vi "UHR-Fleezers Control (fpga) - 9.2.vi"() -> ()   [LabVIEW 2009]
doc: "UHR-Fleezers Instrument Control Code (fpga)"
uses:
  <vilib>/Platform/TimedLoop/XDataNode/XDataNode.xnode
  <vilib>/Platform/TimedLoop/XDataNode/loadlvalarms.vi
  <vilib>/Platform/TimedLoop/XDataNode/timing_clust.ctl
  <vilib>/Platform/TimedLoop/XDataNode/nitl_modes.ctl
  <vilib>/Platform/TimedLoop/XDataNode/wakeup.ctl
  <vilib>/eio/EIONode/EIONode.xnode
  <vilib>/rvi/eio/nirviEIOImplementation/nirviEIOImplementation.xnode
  <vilib>/rvi/eio/common/nirviEmuTemplateMethod_noerrors.vi
  <vilib>/rvi/eio/common/nirviEmuClasses.ctl
  <vilib>/eio/EIOMethodNode/EIOMethodNode.xnode
  <vilib>/rvi/eio/nirviEIOMethodImplementation/nirviEIOMethodImplementation.xnode
  <vilib>/rvi/DataTransferAndStorage/Container/XNode/niFpgaContainer.xnode
  <vilib>/rvi/interface/RandomDataEmulation/niFpgaRandomDataHandleErrors.vi
  <vilib>/rvi/interface/RandomDataEmulation/nirviRandomDataFPGAFIFO.vi
  <vilib>/rvi/DataTransferAndStorage/Container/Common/niFpgaContainerMethod.ctl
  <vilib>/rvi/DataTransferAndStorage/Container/Common/niFpgaTransferTypeControl.ctl
  <vilib>/Platform/TimedLoop/XDataNode/XDNodeRunTimeDep.lvlib
panel:
  in  "Tab Control":T1(tab)=enum."APD Counting"
  in  "AI Averages":u16=1 min=1 step=1
  in  "AI1 Sets to FIFO":T2={"Set 1"=TRUE, "Set 2"=TRUE, "Set 3"=FALSE}
  in  "N of AI1 Int Acq Sets":i16=2 min=1 max=3 step=1
  out "Number of AI channels":i16
  out "AI Late Counter":u32
  in  "ai count":u32=400
  out "AI late?":bool
  in  "+ phase":bool
  in  "Phase count adjustment":i16
  out "Relative phase":i16
  in  "DMA buffer timeout":i32
  in  "AI to FIFO":bool
  in  "Tab Control 2":T3(tab)
  in  "Swap F1 and F2":bool
  in  "Freq or Amp switch first":bool=TRUE
  in  "Cont. Scan":bool
  in  "Abort scan":bool
  in  "Cycles per step":u64
  in  "Scan BD":bool
  in  "Number of scans":u16
  in  "Scan steps":u64
  in  "Scan freq.  increment":i64
  out "Scanning":bool
  in  "Start scan":bool
  in  "OSK Bd 1":bool
  in  "Reset Bd 1":bool
  in  "RD":bool
  in  "PMODE":bool
  in  "OSK Bd 2":bool
  in  "Reset Bd 2":bool
  in  "Direct RF Box \nCommunication":bool
  in  "Data BD 2":u8 format="%08b"
  in  "Data BD 1":u8 format="%08b"
  in  "Address":u8 format="%02x"
  in  "Update Data":bool
  in  "FPGA Controls\n RF Box":bool
  in  "Number Interlace Cycles":u8=2 min=1 max=3
  in  "Interlace Off Parameters":u8=1 min=1 max=3
  in  "Interlace ON/OFF":bool
  out "DIO Relative phase":i16
  in  "Phase count adjustment (DIO)":i16
  in  "+ phase (DIO)":bool
  out "DIO Late Counter":u32
  out "DIO Late?":bool
  in  "DIO count 1 (ticks)":u32=400
  in  "DIO count 2 (ticks)":u32=400
  in  "DIO count 3 (ticks)":u32=400
  out "AI2 Y Sum Set 2":i16
  out "AI2 Y Sum Set 1":i16
  in  "FB Gains Set 1":T4={"proportional gain (Kc)"=10, "integral gain (Kc*Ts/Ti)"=5, "derivative gain (Kc*Td/Ts)"=0}
  in  "FB Setpoint Set 1":i16 min=0 step=1
  in  "FB Reset Set 1":bool
  in  "FB On/Off Set 1":bool
  in  "FB Reset Set 2":bool
  in  "FB On/Off Set 2":bool
  in  "FB Setpoint Set 2":i16 min=0 step=1
  in  "FB Gains Set 2":T4={"proportional gain (Kc)"=10, "integral gain (Kc*Ts/Ti)"=5, "derivative gain (Kc*Td/Ts)"=0}
  in  "FB output range 2":cluster{"output high":i16, "output low":i16}={"output high"=3000, "output low"=0}
  in  "FB output range 1":cluster{"output high":i16, "output low":i16}={"output high"=3000, "output low"=0}
  out "Scan I":u64
  in  "Amp switch delay":u16=5
  in  "Freq switch delay":u16
  in  "BD 2 Amplitude 1":u16
  in  "BD 1 Amplitude 1":u16
  in  "BD 2 Frequency 1":u64
  in  "BD 1 Frequency 1":u64
  in  "BD 2 Amplitude 2":u16
  in  "BD 1 Amplitude 2":u16
  in  "BD 2 Frequency 2":u64
  in  "BD 1 Frequency 2":u64
  in  "BD 2 Amplitude 3":u16
  in  "BD 1 Amplitude 3":u16
  in  "BD 2 Frequency 3":u64
  in  "BD 1 Frequency 3":u64
  out "Numeric":i32
  out "AO2 2":i16
  out "AO1 2":i16
  in  "1D or 2D Scan?":bool
  in  "Abort scan (MCL)":bool
  in  "MCL Scan Axis":bool
  in  "Cont. Scan (MCL)":bool
  out "Scan I (MCL)":u64
  in  "Number of scans (MCL)":u16
  out "Scanning MCL":bool
  in  "Scan steps (MCL)":u64
  in  "Cycles per step (MCL)":u64
  in  "Scan freq.  increment (MCL)":i16
  in  "Start scan (MCL)":bool
  in  "AO2":i16
  in  "AO1":i16
  out "MCL Late Counter":u32
  out "MCL Late?":bool
  in  "MCL count":u32=800
  out "MCL Relative Phase":i16
  in  "Phase count adjustment (MCL)":i16
  in  "+ phase (MCL)":bool
  in  "APD2 Trigger on Edge?":bool=TRUE
  in  "APD1 Trigger on Edge?":bool=TRUE
  in  "APD Gate Operating Mode":u8 max=2 step=1
  in  "Invert APD Gate":bool
  in  "APD Gate OFF Count":u32=100
  in  "APD Gate ON Count":u32=300
  out "APD Gate Late Counter":u32
  out "APD Gate Late?":bool
  out "APD Gate Relative Phase":i16
  in  "Phase count adjustment (APD Gate)":i16
  in  "+ phase (APD Gate)":bool
  out "APD 2 Counts 0":u32
  out "APD 2 Counts 1":u32
  out "APD 1 Counts 0":u32
  out "APD 1 Counts 1":u32
  out "APD out state":bool
  in  "APD 2 AO offset":i16
  in  "APD 1 AO offset":i16
  in  "APD 2 AO scale factor":i16=1
  in  "APD 1 AO scale factor":i16=1
  in  "APD to FIFO":bool
  in  "APD Acq Rate Count":u32=20000000
  out "APD Acq Late Counter":u32
  out "APD Acq Late?":bool
  out "APD Acq Relative Phase":i16
  in  "Phase Count Adjustment (APD Acq)":i16
  in  "+ phase (APD Acq)":bool
  in  "Green Filter Flipper":bool
  out "Green FB Signals":T5
  in  "Green FB Count":u32=1200
  out "Green Late Counter":u32
  out "Green FB Late?":bool
  out "Green FB Relative Phase":i16
  in  "Phase count adjustment (Green FB)":i16=10
  in  "+ phase (Green FB)":bool
  out "Green FB Sum":i16
  in  "Green int current ON count adj":u32=150
  in  "Current Out":u16=30000
  in  "Green FB On/Off":bool
  in  "Green FB Setpoint":i16=250 min=0 step=1
  in  "Green FB Gains":T4={"proportional gain (Kc)"=10, "integral gain (Kc*Ts/Ti)"=5, "derivative gain (Kc*Td/Ts)"=0}
  in  "Green FB Reset":bool
  in  "Operating Mode 2":u8=2 max=2 step=1
  in  "Invert GI 2":bool
  in  "Green interlace OFF count 2":u32=900
  in  "Green interlace ON count 2":u32=300
  out "GI Late Counter 2":u32
  out "GI Late? 2":bool
  out "GI Relative phase 2":i16
  in  "Phase count adjustment (GI) 2":i16=20
  in  "+ phase (GI) 2":bool
  in  "Green interlace OFF count":u32=100
  out "GI Relative phase":i16
  in  "Phase count adjustment (GI)":i16
  in  "+ phase (GI)":bool
  out "GI Late?":bool
  in  "Green interlace ON count":u32=300
  out "GI Late Counter":u32
  in  "Invert GI":bool
  in  "Operating Mode":u8 max=2 step=1
  in  "Connector0/DIO9":bool
  in  "Connector1/DIO32":bool
  in  "Connector1/DIO33":bool
  in  "Connector1/DIO34":bool
  in  "Chassis2/Mod4/AO1":u16
  in  "Extra DO Counts":u32=40000
  # "Only one of these can be on\nat a time:"
  # "Raster Scan AOD"
  # "1 (X)"
  # "2 (Y)"
  # "IR Intensity Feedback (RF BD 1)"
  # "AO1 (Y)"
  # "2D"
  # "1D"
  # "AO2 (X)"
  # "APD AO for aligning"
  # "Detection Loop"
  # "Green fluorescent laser digital gate interlacing loop"
  # "0 Forced ON\n1 Forced OFF\n2 Interlacing"
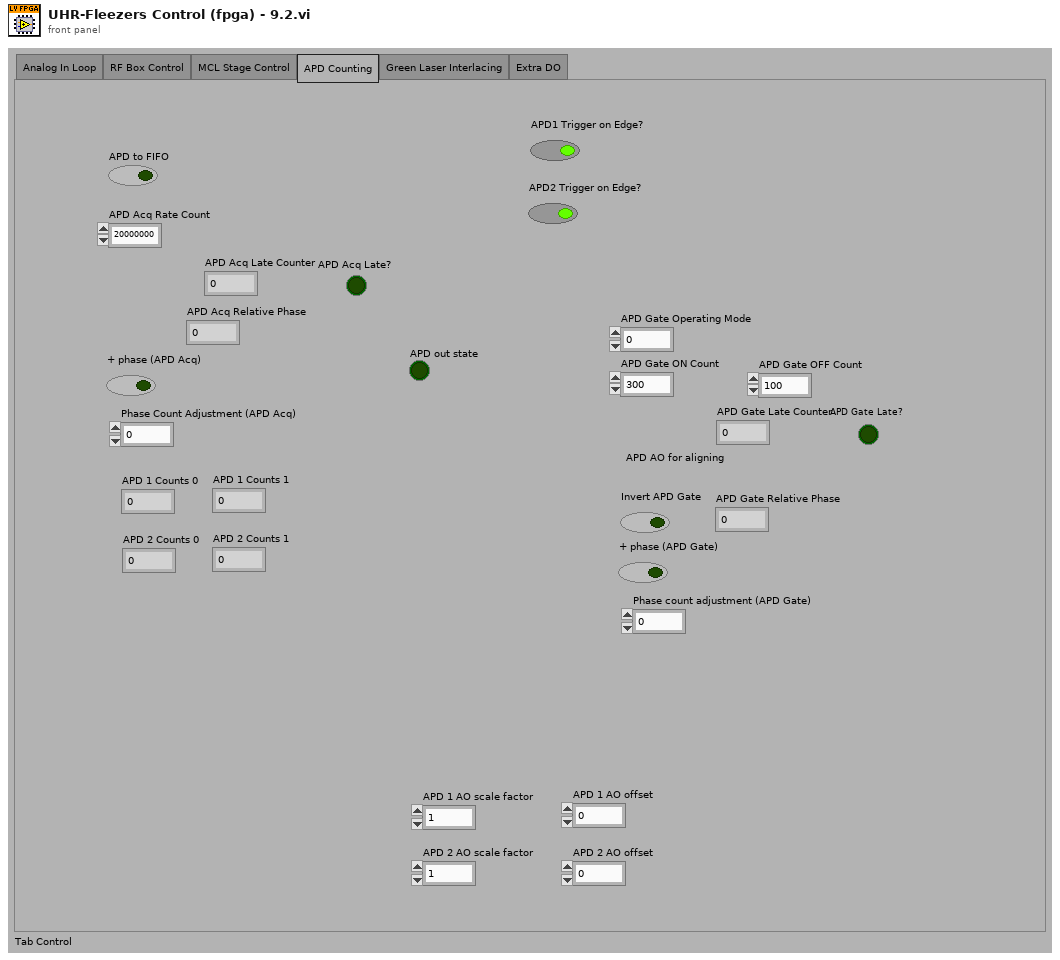
[diagram p1: front panel]
types:
  T1 = enum32{"Analog In Loop", "RF Box Control", "MCL Stage Control", "APD Counting", "Green Laser Interlacing", "Extra DO"}
  T2 = cluster{"Set 1":bool, "Set 2":bool, "Set 3":bool}
  T3 = enum32{"Controls", "Interlacing Frequency and Amplitude Values"}
  T4 = cluster{"proportional gain (Kc)":i16, "integral gain (Kc*Ts/Ti)":i16, "derivative gain (Kc*Td/Ts)":i16}
  T5 = cluster{"Green FB Ch 0":i16, "Green FB Ch 1":i16, "Green FB Ch 2":i16}
  T6 = typedef "nirviEmuClasses.ctl" = enum16{"IO Read", "IO Write", "Method", "Property Read", "Property Write"}
  T7 = typedef "XDNodeRunTimeDep.lvlib/timing_clust.ctl" = cluster{"Expected End [f-1]":u64, "Actual End [f-1]":u64, "Finished Late? [f-1]":bool, "Expected End [i-1]":u64, "Actual End [i-1]":u64, "Finished Late? [i-1]":bool, "Expected Start [i]":u64, "Actual Start [i]":u64, "Expected Start [f]":u64, "Actual Start [f]":u64, "Source Name":string, "Structure Name":string, "Period":i64, "Deadline":i64, "Offset":i64, "Start":i64, "Priority":i32, "Timeout":i32, "Mode":T8, "Wakeup Reason":T9, "Error":errorcluster, "Source Type":string, "Secondary Source Type":string, "Global End Time":u64, "Global Start Time":u64, "Frame Duration":u64, "Iteration Duration":u64, "Assigned CPU":i32, "I/O Scan Engine Mode":u32}
  T8 = typedef "XDNodeRunTimeDep.lvlib/nitl_modes.ctl" = enum32{"No Change", "Process missed periods, maintain original phase", "Discard missed periods, maintain original phase", "Process missed periods, ignore original phase", "Discard missed periods, ignore original phase"}
  T9 = typedef "XDNodeRunTimeDep.lvlib/wakeup.ctl" = enum32{"Normal", "Aborted", "Asynchronous wakeup", "Timing source error", "Timed loop error", "Timeout"}
  T10 = cluster{"Chassis2/Mod1/AI0":i16, "Chassis2/Mod1/AI1":i16, "Chassis2/Mod1/AI2":i16}
  T11 = typedef "niFpgaContainerMethod.ctl" = enum16{"Write", "Read", "Clear", "Get Number of Elements to Write", "Get Number of Elements to Read", "Enable", "Disable", "Flush and Disable", "Get Stream State"}
  T12 = typedef "niFpgaTransferTypeControl.ctl" = enum16{"Target-Scoped", "Host to Target - DMA", "Target to Host - DMA", "Peer to Peer Reader", "Peer to Peer Writer", "Bidirectional"}
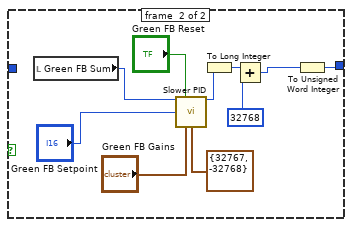
[diagram p2: hidden frame]
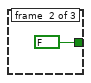
[diagram p3: hidden frame]
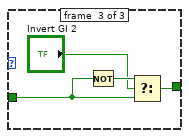
[diagram p4: hidden frame]
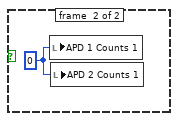
[diagram p5: hidden frame]
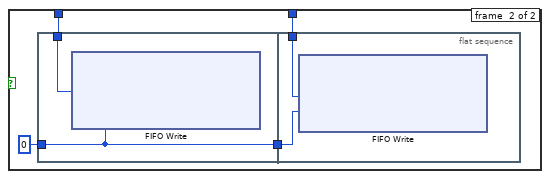
[diagram p6: hidden frame]
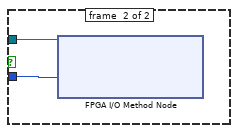
[diagram p7: hidden frame]
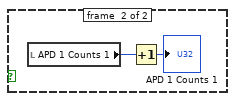
[diagram p8: hidden frame]
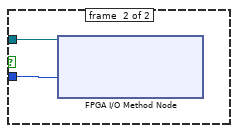
[diagram p9: hidden frame]
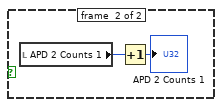
[diagram p10: hidden frame]
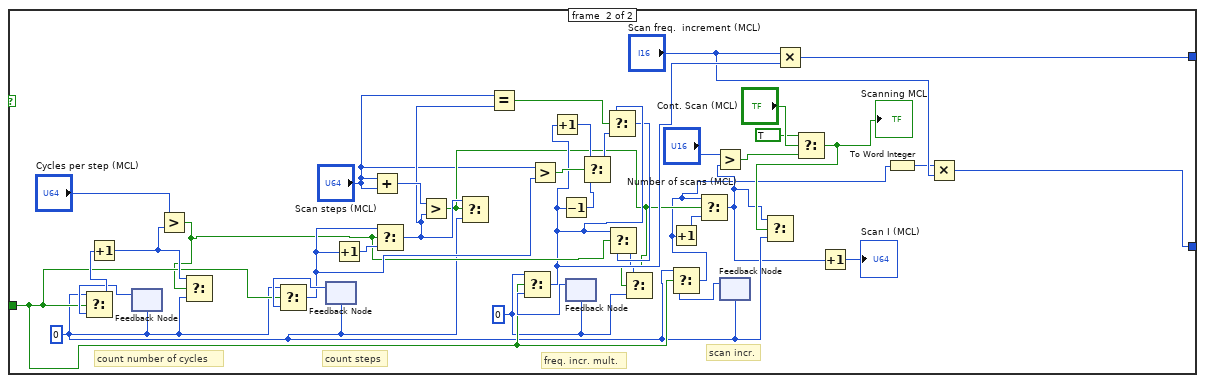
[diagram p11: hidden frame]
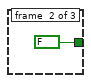
[diagram p12: hidden frame]
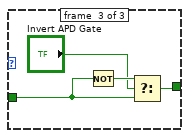
[diagram p13: hidden frame]
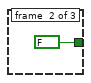
[diagram p14: hidden frame]
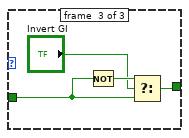
[diagram p15: hidden frame]
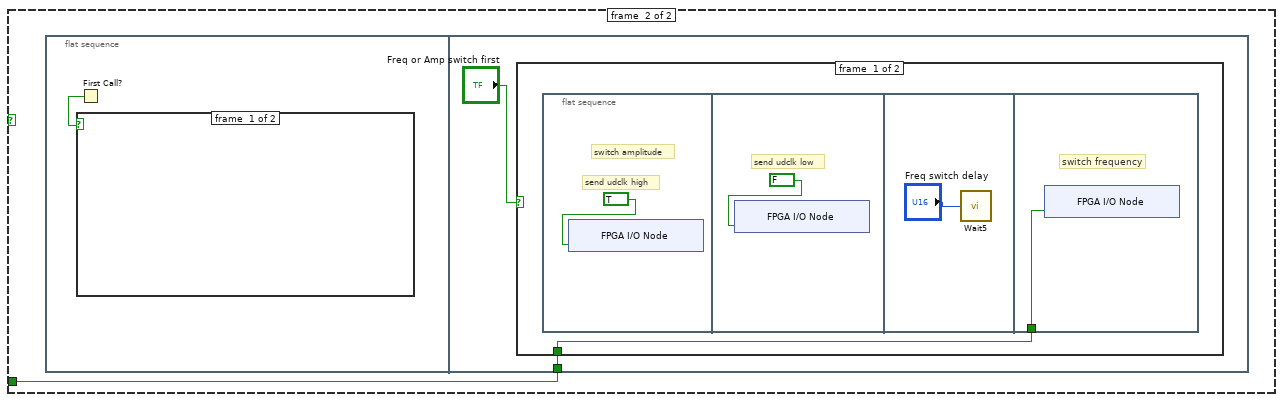
[diagram p16: hidden frame]
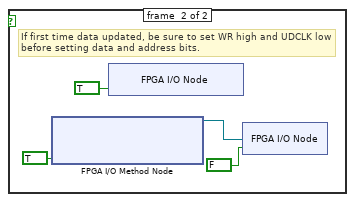
[diagram p17: hidden frame]
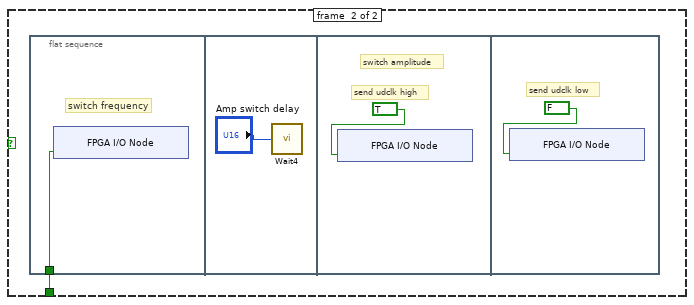
[diagram p18: hidden frame]
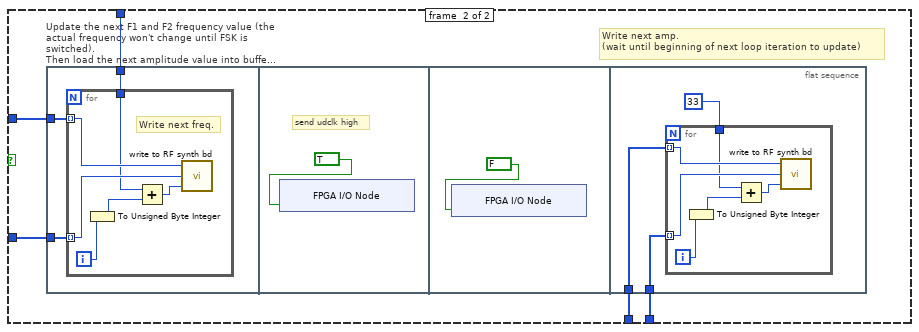
[diagram p19: hidden frame]
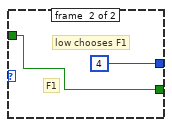
[diagram p20: hidden frame]
diagram:
  # "timing array current index"
  # "timing array"
  # "timing counter (phase adjusted here)"
  # "late counter"
  n1 = flat-sequence "FPGA initialization to do before running any of the loops" {
    tunnel: [u32 0 ("DIO count 3 (ticks)")] -> w1
    tunnel: [w10] -> _
    frame #0 {
      # "This is a kludge to let host programs know how many channels of data are in the DMA stream.  Set by hand."
      # "Start up expansion chassis early\nto avoid delays later"
      # "This pin controls udclk on the RF boards.\nWhen initially configuring the boards, this pin needs to be\nconfigured as a high impedance input.  Later it will be switched\nto an output."
      # "Initial setting of DIO data and \naddress to low (before reset).  \nThis needs to happen before the other\ncontrol method loops execute."
      n2 = xnode "FPGA I/O Node"("Chassis2/Mod4/AO0"=u16 0) -> ("Chassis2/Mod1/AI0"=w10:i16)  [unwired: 2 in, 2 out]
      n3 = xnode "FPGA I/O Method Node"("Enable"=FALSE) -> ()  [unwired: 1 in, 1 out]
      n4 = xnode "FPGA I/O Node"("Connector1/DIO0"=FALSE, "Connector1/DIO1"=FALSE, "Connector1/DIO2"=FALSE, "Connector1/DIO3"=FALSE, "Connector1/DIO4"=FALSE, "Connector1/DIO5"=FALSE, "Connector1/DIO6"=FALSE, "Connector1/DIO7"=FALSE, "Connector1/DIO8"=FALSE, "Connector1/DIO9"=FALSE, "Connector1/DIO10"=FALSE, "Connector1/DIO11"=FALSE, "Connector1/DIO12"=FALSE, "Connector1/DIO13"=FALSE, "Connector1/DIO15"=FALSE, "Connector1/DIO20"=FALSE, "Connector1/DIO21"=FALSE, "Connector1/DIO22"=FALSE, "Connector1/DIO23"=FALSE, "Connector1/DIO24"=FALSE, "Connector1/DIO25"=FALSE, "Connector1/DIO26"=FALSE, "Connector1/DIO27"=FALSE, "Connector1/DIO14"=FALSE) -> ()  [unwired: 24 in, 24 out]
      "Number of AI channels" <- i16 12 ("Number of AI channels")
    }
  }
  n5 = node-c288() -> (w3:T7)  [unwired: 1 in]
  n6 = local read "AO1"() -> (w5:i16)
  n7 = local read "AO2"() -> (w4:i16)
  n8 = timed-loop "RF box board DIO control: control bits" {
    timing: w3 -> [_]
    timing-out: [_] -> w2
    tunnel: [w393] -> _
    tunnel: w1 -> [w393]
    stop <- FALSE stop-if-true
    n9 = xnode "FPGA I/O Node"("Connector1/DIO16"="RD", "Connector1/DIO17"="PMODE", "Connector1/DIO18"="OSK Bd 1", "Connector1/DIO19"="Reset Bd 1", "Connector1/DIO28"="OSK Bd 2", "Connector1/DIO29"="Reset Bd 2") -> ()  [unwired: 6 in, 6 out]
  }
  n10 = while "APD 1 Counter" {
    tunnel: w1 -> [_]
    stop <- FALSE stop-if-true
    n11 = flat-sequence {
      frame #0 {
        n12 = case shown="False" "APD1 Trigger on Edge?" {
          tunnel: refnum<k21> "Connector0/DIO10" ("APD 1 DO") -> [w486 w511]
          tunnel: -1 ("Timeout") -> [w485 w510]
          frame #0 {
            n13 = xnode "FPGA I/O Method Node"("FPGA I/O In"=w486, "Timeout"=w485) -> ()  [unwired: 2 out]
          }
          frame #1 {
            n14 = xnode "FPGA I/O Method Node"("FPGA I/O In"=w511, "Timeout"=w510) -> ()  [unwired: 2 out]
          }
        }
      }
      frame #1 {
        n15 = local read "APD out state"() -> (w535:bool)
        n16 = case shown="False" w535 {
          frame #0 {
            n17 = local read "APD 1 Counts 0"() -> (w537:u32)
            n18 = Increment(x=w537) -> (x+1=→"APD 1 Counts 0":u32)
          }
          frame #1 {
            n19 = local read "APD 1 Counts 1"() -> (w539:u32)
            n20 = Increment(x=w539) -> (x+1=→"APD 1 Counts 1":u32)
          }
        }
      }
    }
  }
  n21 = while "APD 2 Counter" {
    tunnel: w1 -> [_]
    stop <- FALSE stop-if-true
    n22 = flat-sequence {
      frame #0 {
        n23 = case shown="False" "APD2 Trigger on Edge?" {
          tunnel: refnum<k21> "Connector0/DIO11" ("APD 2 DO") -> [w545 w570]
          tunnel: -1 ("Timeout") -> [w544 w569]
          frame #0 {
            n24 = xnode "FPGA I/O Method Node"("FPGA I/O In"=w545, "Timeout"=w544) -> ()  [unwired: 2 out]
          }
          frame #1 {
            n25 = xnode "FPGA I/O Method Node"("FPGA I/O In"=w570, "Timeout"=w569) -> ()  [unwired: 2 out]
          }
        }
      }
      frame #1 {
        n26 = local read "APD out state"() -> (w594:bool)
        n27 = case shown="False" w594 {
          frame #0 {
            n28 = local read "APD 2 Counts 0"() -> (w596:u32)
            n29 = Increment(x=w596) -> (x+1=→"APD 2 Counts 0":u32)
          }
          frame #1 {
            n30 = local read "APD 2 Counts 1"() -> (w598:u32)
            n31 = Increment(x=w598) -> (x+1=→"APD 2 Counts 1":u32)
          }
        }
      }
    }
  }
  n32 = while "APD Gating" {
    shift-right: [w602] -> _
    shift-left: w1 -> [w607]
    shift-right: [w601] -> _
    shift-left: FALSE -> [w599]
    stop <- FALSE stop-if-true
    n33 = flat-sequence {
      tunnel: w607 -> [w610]
      tunnel: [w611] -> w605
      tunnel: [w610] -> w603
      tunnel: [w609] -> w600
      tunnel: w599 -> [w609]
      tunnel: [w614] -> w606
      tunnel: w605 -> [w614]
      tunnel: [w613] -> w604
      tunnel: w603 -> [w613]
      tunnel: w600 -> [w612]
      tunnel: [w724] -> w602
      tunnel: w606 -> [w746]
      tunnel: w604 -> [w743]
      tunnel: [w729] -> w601
      frame #0 {
        n34 = call "Loop Timer7"("Count(Ticks)"=w610) -> ("Tick Count(Ticks)"=w611:u32)
      }
      frame #1 {
        # "Can switch 2 APDs\n(need 4 channels/APD)"
        n35 = xnode "FPGA I/O Node"("Connector0/DIO0"=w612, "Connector0/DIO1"=w612, "Connector0/DIO2"=w612, "Connector0/DIO3"=w612, "Connector0/DIO4"=w612, "Connector0/DIO5"=w612, "Connector0/DIO6"=w612, "Connector0/DIO7"=w612) -> ()  [unwired: 8 in, 8 out]
      }
      frame #2 {
        n36 = feedback #1(TRUE) -> (w732:bool)
        n37 = feedback #2(w746) -> (w745:u32)
        n38 = Not(x=w732) -> (.not. x?=w728:bool)
        n39 = Subtract(x=w746, y=w745) -> (x-y=w744:u32)
        n40 = Select(t="APD Gate ON Count", s=w728, f="APD Gate OFF Count") -> (s? t:f=w734:u32)
        n41 = Subtract(x=w744, y=w743) -> (x-y=w735:u32)
        n42 = Subtract(x=w734, y=w735) -> (x-y=w723:u32)
        n43 = Greater?(x=w735, y=u32 0) -> (0:w739:bool)
        "APD Gate Late?" <- w739
        n44 = Boolean To (0,1)(Boolean="+ phase (APD Gate)") -> (0, 1=w721:i16)
        n45 = Multiply(x=w721, y="Phase count adjustment (APD Gate)") -> (x*y=w719:i16)
        n46 = feedback #3(u32 0) -> (w741:u32)
        n47 = Increment(x=w741) -> (x+1=w740:u32)
        n48 = Select(t=w740, s=w739, f=w741) -> (s? t:f=w738:u32)
        "APD Gate Late Counter" <- w738
        n49 = Add(x=w723, y=w719) -> (x+y=w724:u32)
        n50 = feedback #4(i16 0) -> (w726:i16)
        n51 = Subtract(x=w726, y=w719) -> (x-y=w725:i16)
        "APD Gate Relative Phase" <- w725
        n52 = case shown="2" "APD Gate Operating Mode" {
          tunnel: [TRUE FALSE w752] -> w729
          tunnel: w732 -> [_ _ w749]
          frame #0 {
          }
          frame #1 {
          }
          frame #2 {
            n53 = Not(x=w749) -> (.not. x?=w751:bool)
            n54 = Select(t=w751, s="Invert APD Gate", f=w749) -> (s? t:f=w752:bool)
          }
        }
      }
    }
  }
  n55 = while "Control Additional IO (Green laser flip mount)" {
    stop <- FALSE stop-if-true
    n56 = xnode "FPGA I/O Node"("Connector0/DIO8"="Green Filter Flipper", "Connector0/DIO9"="Connector0/DIO9", "Connector1/DIO32"="Connector1/DIO32", "Connector1/DIO33"="Connector1/DIO33", "Connector1/DIO34"="Connector1/DIO34", "Chassis2/Mod4/AO1"="Chassis2/Mod4/AO1") -> ()  [unwired: 6 in, 6 out]
    n57 = call "Loop Timer2"("Count(Ticks)"="Extra DO Counts") -> ()  [unwired: 1 out]
  }
  n58 = while "Green excitation laser feedback measurement" {
    shift-right: [w827] -> _
    shift-left: w1 -> [w832]
    stop <- FALSE stop-if-true
    n59 = flat-sequence {
      tunnel: w832 -> [w834]
      tunnel: [w835] -> w830
      tunnel: [w834] -> w828
      tunnel: [w842] -> w831
      tunnel: w830 -> [w842]
      tunnel: [w841] -> w829
      tunnel: w828 -> [w841]
      tunnel: [w918] -> w827
      tunnel: w831 -> [w936]
      tunnel: w829 -> [w933]
      frame #0 {
        n60 = call "Loop Timer9"("Count(Ticks)"=w834) -> ("Tick Count(Ticks)"=w835:u32)
      }
      frame #1 {
        n61 = xnode "FPGA I/O Node"("Connector1/DIO35"=TRUE) -> ("Chassis2/Mod1/AI0"=w840:i16, "Chassis2/Mod1/AI1"=w839:i16, "Chassis2/Mod1/AI2"=w836:i16)  [unwired: 4 in, 4 out]
        "Green FB Sum" <- w836
        n62 = Bundle("Chassis2/Mod1/AI0"=w840, "Chassis2/Mod1/AI1"=w839, "Chassis2/Mod1/AI2"=w836) -> (→"Green FB Signals":T10)  [unwired: 1 out]
      }
      frame #2 {
        n63 = feedback #5(w936) -> (w935:u32)
        n64 = Subtract(x=w936, y=w935) -> (x-y=w934:u32)
        n65 = xnode "FPGA I/O Node"("Connector1/DIO35"=FALSE) -> ()  [unwired: 1 in, 1 out]
        n66 = Subtract(x=w934, y=w933) -> (x-y=w927:u32)
        n67 = Subtract(x="Green FB Count", y=w927) -> (x-y=w922:u32)
        n68 = Greater?(x=w927, y=u32 0) -> (0:w929:bool)
        "Green FB Late?" <- w929
        n69 = Boolean To (0,1)(Boolean="+ phase (Green FB)") -> (0, 1=w920:i16)
        n70 = Multiply(x=w920, y="Phase count adjustment (Green FB)") -> (x*y=w915:i16)
        n71 = feedback #6(u32 0) -> (w931:u32)
        n72 = Increment(x=w931) -> (x+1=w930:u32)
        n73 = Select(t=w930, s=w929, f=w931) -> (s? t:f=w928:u32)
        "Green Late Counter" <- w928
        n74 = Add(x=w922, y=w915) -> (x+y=w918:u32)
        n75 = feedback #7(i16 0) -> (w917:i16)
        n76 = Subtract(x=w917, y=w915) -> (x-y=w916:i16)
        "Green FB Relative Phase" <- w916
      }
    }
  }
  n77 = while "Green fluorescent laser interlacing (DO to IA 532 nm AOM ME amp)." {
    shift-right: [w952] -> _
    shift-left: w1 -> [w957]
    shift-right: [w951] -> _
    shift-left: FALSE -> [w949]
    stop <- FALSE stop-if-true
    n78 = flat-sequence {
      tunnel: w957 -> [w960]
      tunnel: [w961] -> w955
      tunnel: [w960] -> w953
      tunnel: [w959] -> w950
      tunnel: w949 -> [w959]
      tunnel: [w964] -> w956
      tunnel: w955 -> [w964]
      tunnel: [w963] -> w954
      tunnel: w953 -> [w963]
      tunnel: w950 -> [w962]
      tunnel: [w1004] -> w952
      tunnel: w956 -> [w1031]
      tunnel: w954 -> [w1028]
      tunnel: [w1014] -> w951
      frame #0 {
        n79 = call "Loop Timer4"("Count(Ticks)"=w960) -> ("Tick Count(Ticks)"=w961:u32)
      }
      frame #1 {
        n80 = xnode "FPGA I/O Node"("Connector1/DIO37"=w962, "Connector1/DIO38"=w962, "Connector1/DIO39"=w962) -> ()  [unwired: 3 in, 3 out]
      }
      frame #2 {
        n81 = feedback #8(w1031) -> (w1030:u32)
        n82 = Subtract(x=w1031, y=w1030) -> (x-y=w1029:u32)
        n83 = Subtract(x=w1029, y=w1028) -> (x-y=w1020:u32)
        n84 = Greater?(x=w1020, y=u32 0) -> (0:w1024:bool)
        "GI Late?" <- w1024
        n85 = Boolean To (0,1)(Boolean="+ phase (GI)") -> (0, 1=w1009:i16)
        n86 = Multiply(x=w1009, y="Phase count adjustment (GI)") -> (x*y=w1006:i16)
        n87 = feedback #9(u32 0) -> (w1026:u32)
        n88 = Increment(x=w1026) -> (x+1=w1025:u32)
        n89 = Select(t=w1025, s=w1024, f=w1026) -> (s? t:f=w1023:u32)
        "GI Late Counter" <- w1023
        n90 = feedback #10(i16 0) -> (w1007:i16)
        n91 = Subtract(x=w1007, y=w1006) -> (x-y=w1005:i16)
        "GI Relative phase" <- w1005
        n92 = feedback #11(TRUE) -> (w1017:bool)
        n93 = case shown="2" "Operating Mode" {
          tunnel: [TRUE FALSE w1037] -> w1014
          tunnel: w1017 -> [_ _ w1034]
          frame #0 {
          }
          frame #1 {
          }
          frame #2 {
            n94 = Not(x=w1034) -> (.not. x?=w1036:bool)
            n95 = Select(t=w1036, s="Invert GI", f=w1034) -> (s? t:f=w1037:bool)
          }
        }
        n96 = Not(x=w1017) -> (.not. x?=w1013:bool)
        n97 = Select(t="Green interlace ON count", s=w1013, f="Green interlace OFF count") -> (s? t:f=w1019:u32)
        n98 = Subtract(x=w1019, y=w1020) -> (x-y=w1010:u32)
        n99 = Add(x=w1010, y=w1006) -> (x+y=w1004:u32)
      }
    }
  }
  n100 = while "Green fluorescent laser interlacing (Current to IA 532 nm AOM ME amp)." {
    shift-right: [w1043] -> _
    shift-left: w1 -> [w1046]
    shift-right: [w1040] -> _
    shift-left: w1 -> [w1038]
    stop <- FALSE stop-if-true
    n101 = flat-sequence {
      tunnel: w1046 -> [w1049]
      tunnel: [w1050] -> w1045
      tunnel: [w1049] -> w1044
      tunnel: [w1048] -> w1039
      tunnel: w1038 -> [w1048]
      tunnel: [w1053] -> w1042
      tunnel: w1045 -> [w1053]
      tunnel: [w1052] -> w1041
      tunnel: w1044 -> [w1052]
      tunnel: w1039 -> [w1051]
      tunnel: [w1066] -> w1043
      tunnel: [w1084] -> w1040
      tunnel: w1042 -> [w1103]
      tunnel: w1041 -> [w1100]
      frame #0 {
        n102 = call "Loop Timer10"("Count(Ticks)"=w1049) -> ("Tick Count(Ticks)"=w1050:u32)
      }
      frame #1 {
        n103 = xnode "FPGA I/O Node"("Chassis2/Mod4/AO0"=w1051) -> ()  [unwired: 1 in, 1 out]
      }
      frame #2 {
        n104 = Subtract(x="Green interlace OFF count 2", y="Green int current ON count adj") -> (x-y=w1076:u32)
        n105 = feedback #12(w1103) -> (w1102:u32)
        n106 = Add(x="Green int current ON count adj", y="Green interlace ON count 2") -> (x+y=w1077:u32)
        n107 = Subtract(x=w1103, y=w1102) -> (x-y=w1101:u32)
        n108 = Subtract(x=w1101, y=w1100) -> (x-y=w1092:u32)
        n109 = Greater?(x=w1092, y=u32 0) -> (0:w1096:bool)
        "GI Late? 2" <- w1096
        n110 = Boolean To (0,1)(Boolean="+ phase (GI) 2") -> (0, 1=w1072:i16)
        n111 = Multiply(x=w1072, y="Phase count adjustment (GI) 2") -> (x*y=w1068:i16)
        n112 = feedback #13(u32 0) -> (w1098:u32)
        n113 = Increment(x=w1098) -> (x+1=w1097:u32)
        n114 = Select(t=w1097, s=w1096, f=w1098) -> (s? t:f=w1095:u32)
        "GI Late Counter 2" <- w1095
        n115 = feedback #14(i16 0) -> (w1069:i16)
        n116 = Subtract(x=w1069, y=w1068) -> (x-y=w1067:i16)
        "GI Relative phase 2" <- w1067
        n117 = feedback #15(TRUE) -> (w1089:bool)
        n118 = case shown="2" "Operating Mode 2" {
          tunnel: [TRUE FALSE w1120] -> w1078
          tunnel: w1089 -> [_ _ w1117]
          frame #0 {
          }
          frame #1 {
          }
          frame #2 {
            n119 = Not(x=w1117) -> (.not. x?=w1119:bool)
            n120 = Select(t=w1119, s="Invert GI 2", f=w1117) -> (s? t:f=w1120:bool)
          }
        }
        n121 = And(x=w1078, y="Green FB On/Off") -> (x .and. y?=w1079:bool)
        n122 = case shown="True" w1079 {
          tunnel: "Current Out" -> [w1104 _]
          tunnel: [w1104 w1109] -> w1083
          frame #0 {
          }
          frame #1 {
            n123 = local read "Green FB Sum"() -> (w1105:i16)
            n124 = call "Slower PID.vi"("process variable"=w1105, "reset?"="Green FB Reset", "setpoint"="Green FB Setpoint", "PID gains (x 2^8)"="Green FB Gains", "output range"=cluster{"output high":i16, "output low":i16} {"output high"=32767, "output low"=-32768} ("Green FB output range")) -> ("output"=w1113:i16)  [unwired: 10 out]
            n125 = To Long Integer(number=w1113) -> (32bit integer=w1106:i32)
            n126 = Add(x=w1106, y=32768) -> (x+y=w1108:i32)
            n127 = To Unsigned Word Integer(number=w1108) -> (unsigned 16bit integer=w1109:u16)
          }
        }
        n128 = Not(x=w1089) -> (.not. x?=w1086:bool)
        n129 = Select(t=w1077, s=w1086, f=w1076) -> (s? t:f=w1091:u32)
        n130 = Subtract(x=w1091, y=w1092) -> (x-y=w1070:u32)
        n131 = Add(x=w1070, y=w1068) -> (x+y=w1066:u32)
        n132 = Boolean To (0,1)(Boolean=w1078) -> (0, 1=w1085:i16)
        n133 = To Unsigned Word Integer(number=w1085) -> (unsigned 16bit integer=w1082:u16)
        n134 = Multiply(x=w1082, y=w1083) -> (x*y=w1084:u16)
      }
    }
  }
  n135 = while "DAQ AI set 1" {
    shift-right: [w1121] -> _
    shift-left: w1 -> [w1126]
    stop <- FALSE stop-if-true
    n136 = flat-sequence {
      tunnel: w1126 -> [w1136]
      tunnel: [w1137] -> w1124
      tunnel: [w1136] -> w1123
      tunnel: [w1147] -> w1134
      tunnel: [w1146] -> w1133
      tunnel: [w1145] -> w1132
      tunnel: [w1144] -> w1131
      tunnel: [w1143] -> w1130
      tunnel: [w1142] -> w1129
      tunnel: [w1141] -> w1128
      tunnel: [w1140] -> w1127
      tunnel: [w1139] -> w1125
      tunnel: w1124 -> [w1139]
      tunnel: w1123 -> [w1138]
      tunnel: [w1138] -> w1122
      tunnel: [w1324] -> w1121
      tunnel: w1134 -> [w1362]
      tunnel: w1133 -> [w1361]
      tunnel: w1132 -> [w1345]
      tunnel: w1131 -> [w1360]
      tunnel: w1130 -> [w1349]
      tunnel: w1129 -> [w1348]
      tunnel: w1128 -> [w1347]
      tunnel: w1127 -> [w1346]
      tunnel: w1125 -> [w1341]
      tunnel: w1122 -> [w1338]
      frame #0 {
        n137 = call "Loop Timer3"("Count(Ticks)"=w1136) -> ("Tick Count(Ticks)"=w1137:u32)
      }
      frame #1 {
        n138 = xnode "FPGA I/O Node"("Connector1/DIO31"=TRUE ("Connector1/DIO33")) -> ("Connector0/AI0"=w1147:i16, "Connector0/AI1"=w1146:i16, "Connector0/AI2"=w1145:i16, "Connector0/AI3"=w1144:i16, "Connector0/AI4"=w1143:i16, "Connector0/AI5"=w1142:i16, "Connector0/AI6"=w1141:i16, "Connector0/AI7"=w1140:i16)  [unwired: 9 in, 9 out]
      }
      frame #2 {
        # "Adjust phase after data acquired if button pressed"
        n139 = feedback #16(i16 1) -> (w1353:i16)
        n140 = Increment(x=w1353) -> (x+1=w1359:i16)
        n141 = Greater?(x=w1359, y="N of AI1 Int Acq Sets") -> (0:w1356:bool)
        n142 = Select(t=i16 1, s=w1356, f=w1359) -> (s? t:f=w1358:i16)
        n143 = feedback #17(FALSE ("AI to FIFO")) -> (w1343:bool)
        n144 = case shown="1, Default" w1353 {
          tunnel: w1345 -> [w1365 w1369 _]
          tunnel: "AI1 Sets to FIFO" -> [w1367 w1371 w1374]
          tunnel: [w1366 w1370 w1373] -> w1350
          tunnel: ["AI to FIFO" w1368 w1372] -> w1342
          tunnel: w1343 -> [_ w1368 w1372]
          frame #0 {
            n145 = Unbundle By Name(w1367) -> ("Set 1"=w1366:bool)
            "AI2 Y Sum Set 1" <- w1365
          }
          frame #1 {
            n146 = Unbundle By Name(w1371) -> ("Set 2"=w1370:bool)
            "AI2 Y Sum Set 2" <- w1369
          }
          frame #2 {
            n147 = Unbundle By Name(w1374) -> ("Set 3"=w1373:bool)
          }
        }
        n148 = And(x=w1350, y=w1342) -> (x .and. y?=w1352:bool)
        n149 = case shown="True" w1352 {
          tunnel: w1362 -> [_ w1379]
          tunnel: w1361 -> [_ w1380]
          tunnel: w1345 -> [_ w1381]
          tunnel: w1360 -> [_ w1382]
          tunnel: w1349 -> [_ w1386]
          tunnel: w1348 -> [_ w1385]
          tunnel: w1347 -> [_ w1384]
          tunnel: w1346 -> [_ w1383]
          frame #0 {
          }
          frame #1 {
            n150 = Greater?(x="AI Averages", y=u16 1) -> (0:w1377:bool)
            n151 = case shown="True" w1377 {
              tunnel: w1386 -> [w1397 w1454]
              tunnel: w1385 -> [w1396 w1453]
              tunnel: w1384 -> [w1395 w1452]
              tunnel: w1383 -> [w1394 w1451]
              tunnel: w1382 -> [w1393 w1450]
              tunnel: w1381 -> [w1398 w1449]
              tunnel: w1380 -> [w1399 w1448]
              tunnel: w1379 -> [w1400 w1447]
              tunnel: "AI Averages" -> [_ w1434]
              tunnel: "DMA buffer timeout" -> [w1388 w1431]
              frame #0 {
                n152 = Join Numbers(hi=w1400, lo=w1399) -> ((hi.lo)=w1392:u32)
                n153 = Join Numbers(hi=w1398, lo=w1393) -> ((hi.lo)=w1391:u32)
                n154 = Join Numbers(hi=w1397, lo=w1396) -> ((hi.lo)=w1390:u32)
                n155 = Join Numbers(hi=w1395, lo=w1394) -> ((hi.lo)=w1389:u32)
                n156 = Build Array(w1392, w1391, w1390, w1389) -> (w1387:u32[])
                n157 = for {
                  tunnel: w1387 -> [w1402] mode=indexing
                  tunnel: w1388 -> [w1403]
                  n158 = To Unsigned Long Integer(number=w1402) -> (unsigned 32bit integer=w1401:u32)
                  n159 = xnode ("FIFO Write")("Element"=w1401, "Timeout"=w1403) -> ()  [unwired: 1 in, 2 out]
                }
              }
              frame #1 {
                w1438 = u16 0
                n160 = To Long Integer(number=w1447) -> (32bit integer=w1440:i32)
                n161 = To Long Integer(number=w1448) -> (32bit integer=w1457:i32)
                n162 = To Long Integer(number=w1449) -> (32bit integer=w1456:i32)
                n163 = To Long Integer(number=w1450) -> (32bit integer=w1455:i32)
                n164 = To Long Integer(number=w1454) -> (32bit integer=w1446:i32)
                n165 = To Long Integer(number=w1453) -> (32bit integer=w1445:i32)
                n166 = To Long Integer(number=w1452) -> (32bit integer=w1444:i32)
                n167 = To Long Integer(number=w1451) -> (32bit integer=w1443:i32)
                n168 = Build Array(w1440, w1457, w1456, w1455, w1446, w1445, w1444, w1443) -> (w1429:i32[])
                n169 = feedback #18(w1429) -> (w1442:i32[])
                n170 = Add(x=w1429, y=w1442) -> (x+y=w1441:i32[])
                n171 = feedback #19(w1438) -> (w1436:u16)
                n172 = Increment(x=w1436) -> (x+1=w1433:u16)
                n173 = Equal?(x=w1433, y=u16 1) -> (x = y?=w1432:bool)
                n174 = Select(t=w1429, s=w1432, f=w1441) -> (s? t:f=w1430:i32[])
                n175 = Greater Or Equal?(x=w1433, y=w1434) -> (x >= y?=w1435:bool)
                n176 = Select(t=w1438, s=w1435, f=w1433) -> (s? t:f=w1437:u16)
                n177 = case shown="True" w1435 {
                  tunnel: w1430 -> [_ w1459]
                  tunnel: w1431 -> [_ w1458]
                  frame #0 {
                  }
                  frame #1 {
                    n178 = for {
                      tunnel: w1459 -> [w1461] mode=indexing
                      tunnel: w1458 -> [w1462]
                      n179 = To Unsigned Long Integer(number=w1461) -> (unsigned 32bit integer=w1460:u32)
                      n180 = xnode ("FIFO Write")("Element"=w1460, "Timeout"=w1462) -> ()  [unwired: 1 in, 2 out]
                    }
                  }
                }
              }
            }
          }
        }
        n181 = feedback #20(w1341) -> (w1340:u32)
        n182 = Subtract(x=w1341, y=w1340) -> (x-y=w1339:u32)
        n183 = Subtract(x=w1339, y=w1338) -> (x-y=w1335:u32)
        n184 = Subtract(x="ai count", y=w1335) -> (x-y=w1325:u32)
        n185 = Greater?(x=w1335, y=u32 0) -> (0:w1333:bool)
        "AI late?" <- w1333
        n186 = feedback #21(u32 0) -> (w1331:u32)
        n187 = Increment(x=w1331) -> (x+1=w1330:u32)
        n188 = Select(t=w1330, s=w1333, f=w1331) -> (s? t:f=w1332:u32)
        "AI Late Counter" <- w1332
        n189 = xnode "I/O Node"("Connector1/DIO31"=FALSE ("Connector1/DIO34")) -> ()  [unwired: 1 in, 1 out]
        n190 = Boolean To (0,1)(Boolean="+ phase") -> (0, 1=w1327:i16)
        n191 = Multiply(x=w1327, y="Phase count adjustment") -> (x*y=w1321:i16)
        n192 = feedback #22(i16 0) -> (w1323:i16)
        n193 = Add(x=w1325, y=w1321) -> (x+y=w1324:u32)
        n194 = Subtract(x=w1323, y=w1321) -> (x-y=w1322:i16)
        "Relative phase" <- w1322
      }
    }
  }
  n195 = while "RF box board DIO control: parallel communication" {
    shift-right: [w1507] -> _
    shift-left: w1 -> [w1506]
    shift-right: [w1505] -> _
    shift-left: FALSE ("Swap F1 and F2") -> [w1504]
    stop <- FALSE stop-if-true
    n196 = flat-sequence {
      tunnel: w1504 -> [w1511]
      tunnel: w1506 -> [w1509]
      tunnel: [w1511] -> w1503
      tunnel: [w1510] -> w1502
      tunnel: [w1509] -> w1501
      tunnel: [w1517] -> w1507
      tunnel: [w1516] -> w1505
      tunnel: w1503 -> [w1515]
      tunnel: w1502 -> [w1513]
      tunnel: w1501 -> [w1512]
      frame #0 {
        n197 = call "Loop Timer"("Count(Ticks)"=w1509) -> ("Tick Count(Ticks)"=w1510:u32)
      }
      frame #1 {
        n198 = flat-sequence {
          tunnel: ["FPGA Controls\n RF Box"] -> w1514
          tunnel: w1515 -> [w1518]
          tunnel: [w1667] -> w1517
          tunnel: [w1687] -> w1516
          tunnel: w1514 -> [w1686]
          tunnel: w1513 -> [w1680]
          tunnel: w1512 -> [w1677]
          frame #0 {
            n199 = case shown="True" "FPGA Controls\n RF Box" {
              tunnel: w1518 -> [_ w1520]
              frame #0 {
              }
              frame #1 {
                n200 = flat-sequence {
                  tunnel: w1520 -> [w1565]
                  frame #0 {
                    n201 = First Call?() -> (First Call?: T/F=w1521:bool)
                    n202 = case shown="True" w1521 {
                      frame #0 {
                      }
                      frame #1 {
                        # "If first time data updated, be sure to set WR high and UDCLK low\nbefore setting data and address bits."
                        n203 = xnode "FPGA I/O Method Node"("Enable"=TRUE) -> ("FPGA I/O Out"=w1523:refnum<k21>)  [unwired: 1 in]
                        n204 = xnode "FPGA I/O Node"("Connector1/DIO15"=TRUE) -> ()  [unwired: 1 in, 1 out]
                        n205 = xnode "FPGA I/O Node"("I/O Item"=FALSE ("Connector1/DIO30"), "FPGA I/O In"=w1523) -> ()  [unwired: 1 out]
                      }
                    }
                  }
                  frame #1 {
                    n206 = case shown="True" "Freq or Amp switch first" {
                      tunnel: w1565 -> [w1567 w1611]
                      frame #0 {
                        n207 = flat-sequence {
                          tunnel: w1567 -> [w1597]
                          frame #0 {
                            # "switch amplitude"
                            # "send udclk high"
                            n208 = xnode "FPGA I/O Node"("Connector1/DIO30"=TRUE ("Connector1/DIO15")) -> ()  [unwired: 1 in, 1 out]
                          }
                          frame #1 {
                            # "send udclk low"
                            n209 = xnode "FPGA I/O Node"("Connector1/DIO30"=FALSE ("Connector1/DIO15")) -> ()  [unwired: 1 in, 1 out]
                          }
                          frame #2 {
                            n210 = call "Wait5"("Count(Ticks)"="Freq switch delay") -> ()  [unwired: 1 out]
                          }
                          frame #3 {
                            # "switch frequency"
                            n211 = xnode "FPGA I/O Node"("Connector1/DIO36"=w1597) -> ()  [unwired: 1 in, 1 out]
                          }
                        }
                      }
                      frame #1 {
                        n212 = flat-sequence {
                          tunnel: w1611 -> [w1612]
                          frame #0 {
                            # "switch frequency"
                            n213 = xnode "FPGA I/O Node"("Connector1/DIO36"=w1612) -> ()  [unwired: 1 in, 1 out]
                          }
                          frame #1 {
                            n214 = call "Wait4"("Count(Ticks)"="Amp switch delay") -> ()  [unwired: 1 out]
                          }
                          frame #2 {
                            # "switch amplitude"
                            # "send udclk high"
                            n215 = xnode "FPGA I/O Node"("Connector1/DIO30"=TRUE ("Connector1/DIO15")) -> ()  [unwired: 1 in, 1 out]
                          }
                          frame #3 {
                            # "send udclk low"
                            n216 = xnode "FPGA I/O Node"("Connector1/DIO30"=FALSE ("Connector1/DIO15")) -> ()  [unwired: 1 in, 1 out]
                          }
                        }
                      }
                    }
                  }
                }
              }
            }
          }
          frame #1 {
            # "This is the prior cycle's on time"
            # "increment timing\nindex, reset to 0 if \nend of matrix"
            # "Reset to begginning (1) when number of cycles reached."
            # "timing index"
            # "build byte stacks for writing data\n(must correspond to addresses array constant)"
            # "Timing housekeeping"
            # "Adjust phase if late\n(maintains constant phase relationship between cycles)"
            n217 = feedback #23(u8 0 ("t")) -> (w1683:u8)
            n218 = Increment(x=w1683) -> (x+1=w1727:u8)
            n219 = Increment(x="Number Interlace Cycles") -> (x+1=w1722:u8)
            n220 = Equal?(x=w1727, y=w1722) -> (x = y?=w1729:bool)
            n221 = Select(t=u8 1, s=w1729, f=w1727) -> (s? t:f=w1682:u8)
            n222 = Increment(x=w1682) -> (x+1=w1724:u8)
            n223 = Equal?(x=w1724, y=w1722) -> (x = y?=w1725:bool)
            n224 = Select(t=u8 1, s=w1725, f=w1724) -> (s? t:f=w1721:u8)
            n225 = Select(t=w1721, s="Interlace ON/OFF", f="Interlace Off Parameters") -> (s? t:f=w1705:u8)
            n226 = case shown="1, Default" w1705 {
              tunnel: [w1801 "BD 1 Frequency 2" "BD 1 Frequency 3"] -> w1717
              tunnel: [w1800 "BD 2 Frequency 2" "BD 2 Frequency 3"] -> w1706
              tunnel: ["BD 2 Amplitude 1" "BD 2 Amplitude 2" "BD 2 Amplitude 3"] -> w1655
              tunnel: [w1789 w1859 "BD 1 Amplitude 3"] -> w1658
              frame #0 {
                w1796 = u8 0 ("f")
                n227 = local read "Scanning"() -> (w1802:bool)
                n228 = Or(x=w1802, y="Start scan") -> (x .or. y?=w1794:bool)
                n229 = Not(x="Abort scan") -> (.not. x?=w1792:bool)
                n230 = And(x=w1792, y=w1794) -> (x .and. y?=w1791:bool)
                n231 = case "Raster scan" shown="True" w1791 {
                  tunnel: [i16 0 w1848] -> w1797
                  tunnel: "Start scan" -> [_ w1833]
                  frame #0 {
                    n232 = local write "Scanning"(FALSE ("scanning")) -> ()
                  }
                  frame #1 {
                    w1817 = i64 0
                    w1816 = u64 0
                    # "scan incr."
                    # "freq. incr. mult."
                    # "count steps"
                    # "count number of cycles"
                    n233 = feedback #24(w1816) -> (w1845:u64)
                    n234 = Select(t=w1816, s=w1833, f=w1845) -> (s? t:f=w1847:u64)
                    n235 = Increment(x=w1847) -> (x+1=w1844:u64)
                    n236 = Greater?(x="Cycles per step", y=w1844) -> (0:w1826:bool)
                    n237 = Select(t=w1844, s=w1826, f=w1816) -> (s? t:f=w1843:u64)
                    n238 = feedback #25(w1816) -> (w1842:u64)
                    n239 = Select(t=w1816, s=w1833, f=w1842) -> (s? t:f=w1837:u64)
                    n240 = Increment(x=w1837) -> (x+1=w1841:u64)
                    n241 = Add(x="Scan steps", y="Scan steps") -> (x+y=w1840:u64)
                    n242 = Select(t=w1837, s=w1826, f=w1841) -> (s? t:f=w1821:u64)
                    n243 = Greater?(x=w1840, y=w1821) -> (0:w1820:bool)
                    n244 = Select(t=w1821, s=w1820, f=w1816) -> (s? t:f=w1838:u64)
                    n245 = Equal?(x="Scan steps", y=w1821) -> (x = y?=w1825:bool)
                    n246 = Greater?(x="Scan steps", y=w1837) -> (0:w1836:bool)
                    n247 = feedback #26(w1817) -> (w1839:i64)
                    n248 = Select(t=w1817, s=w1833, f=w1839) -> (s? t:f=w1823:i64)
                    n249 = Increment(x=w1823) -> (x+1=w1835:i64)
                    n250 = Decrement(x=w1823) -> (x-1=w1834:i64)
                    n251 = Select(t=w1835, s=w1836, f=w1834) -> (s? t:f=w1824:i64)
                    n252 = Select(t=w1823, s=w1825, f=w1824) -> (s? t:f=w1822:i64)
                    n253 = Select(t=w1823, s=w1826, f=w1822) -> (s? t:f=w1818:i64)
                    n254 = Select(t=w1818, s=w1820, f=w1817) -> (s? t:f=w1819:i64)
                    n255 = feedback #27(w1816) -> (w1832:u64)
                    n256 = Select(t=w1816, s=w1833, f=w1832) -> (s? t:f=w1828:u64)
                    n257 = Increment(x=w1828) -> (x+1=w1829:u64)
                    n258 = Select(t=w1828, s=w1820, f=w1829) -> (s? t:f=w1827:u64)
                    n259 = Greater?(x="Number of scans", y=w1827) -> (0:w1813:bool)
                    n260 = Multiply(x="Scan freq.  increment", y=w1823) -> (x*y=w1848:i64)
                    n261 = Select(t=TRUE, s="Cont. Scan", f=w1813) -> (s? t:f=w1812:bool)
                    "Scanning" <- w1812
                    n262 = Select(t=w1827, s=w1812, f=w1816) -> (s? t:f=w1830:u64)
                    n263 = Increment(x=w1827) -> (x+1=→"Scan I":u64)
                  }
                }
                n264 = case shown="True" "FB On/Off Set 1" {
                  tunnel: "BD 1 Amplitude 1" -> [w1850 _]
                  tunnel: [w1850 w1851] -> w1789
                  frame #0 {
                  }
                  frame #1 {
                    n265 = local read "AI2 Y Sum Set 1"() -> (w1853:i16)
                    n266 = call "Slower PID.vi"("process variable"=w1853, "reset?"="FB Reset Set 1", "setpoint"="FB Setpoint Set 1", "PID gains (x 2^8)"="FB Gains Set 1", "output range"="FB output range 1") -> ("output"=w1856:i16)  [unwired: 10 out]
                    n267 = To Unsigned Word Integer(number=w1856) -> (unsigned 16bit integer=w1851:u16)
                  }
                }
                n268 = Select(t=w1796, s="Scan BD", f=w1797) -> (s? t:f=w1795:i64)
                n269 = Select(t=w1797, s="Scan BD", f=w1796) -> (s? t:f=w1798:i64)
                n270 = Add(x=w1795, y="BD 2 Frequency 1") -> (x+y=w1800:u64)
                n271 = Add(x="BD 1 Frequency 1", y=w1798) -> (x+y=w1801:u64)
              }
              frame #1 {
                n272 = case shown="True" "FB On/Off Set 2" {
                  tunnel: [w1864 w1865] -> w1859
                  tunnel: "BD 1 Amplitude 2" -> [w1864 _]
                  frame #0 {
                  }
                  frame #1 {
                    n273 = local read "AI2 Y Sum Set 2"() -> (w1870:i16)
                    n274 = call "Slower PID.vi"("process variable"=w1870, "reset?"="FB Reset Set 2", "setpoint"="FB Setpoint Set 2", "PID gains (x 2^8)"="FB Gains Set 2", "output range"="FB output range 2") -> ("output"=w1867:i16)  [unwired: 10 out]
                    n275 = To Unsigned Word Integer(number=w1867) -> (unsigned 16bit integer=w1865:u16)
                  }
                }
              }
              frame #2 {
              }
            }
            n276 = feedback #28(w1680) -> (w1679:u32)
            n277 = Subtract(x=w1680, y=w1679) -> (x-y=w1678:u32)
            n278 = Select(t=w1682, s="Interlace ON/OFF", f="Interlace Off Parameters") -> (s? t:f=w1720:u8)
            n279 = Subtract "The error"(x=w1678, y=w1677) -> (x-y=w1675:u32)
            n280 = case shown="3" w1720 {
              tunnel: ["DIO count 1 (ticks)" "DIO count 2 (ticks)" "DIO count 3 (ticks)"] -> w1676
              frame #0 {
              }
              frame #1 {
              }
              frame #2 {
              }
            }
            n281 = Greater?(x=w1675, y=u32 0) -> (0:w1670:bool)
            "DIO Late?" <- w1670
            n282 = feedback #29(u32 0) -> (w1672:u32)
            n283 = Increment(x=w1672) -> (x+1=w1671:u32)
            n284 = Select(t=w1671, s=w1670, f=w1672) -> (s? t:f=w1673:u32)
            "DIO Late Counter" <- w1673
            n285 = Subtract(x=w1676, y=w1675) -> (x-y=w1668:u32)
            n286 = Boolean To (0,1)(Boolean="+ phase (DIO)") -> (0, 1=w1665:i16)
            n287 = Multiply(x=w1665, y="Phase count adjustment (DIO)") -> (x*y=w1661:i16)
            n288 = feedback #30(i16 0) -> (w1663:i16)
            n289 = Subtract(x=w1663, y=w1661) -> (x-y=w1662:i16)
            "DIO Relative phase" <- w1662
            n290 = Split Number(x=w1706) -> (hi(x)=w1711:u32, lo(x)=w1710:u32)
            n291 = Split Number(x=w1717) -> (hi(x)=w1716:u32, lo(x)=w1715:u32)
            n292 = Split Number(x=w1711) -> (lo(x)=w1709:u16)  [unwired: 1 out]
            n293 = Split Number(x=w1710) -> (hi(x)=w1708:u16, lo(x)=w1707:u16)
            n294 = Split Number(x=w1716) -> (lo(x)=w1714:u16)  [unwired: 1 out]
            n295 = Split Number(x=w1715) -> (hi(x)=w1713:u16, lo(x)=w1712:u16)
            n296 = Split Number(x=w1658) -> (hi(x)=w1660:u8, lo(x)=w1659:u8)
            n297 = Split Number(x=w1709) -> (hi(x)=w1697:u8, lo(x)=w1696:u8)
            n298 = Split Number(x=w1708) -> (hi(x)=w1695:u8, lo(x)=w1694:u8)
            n299 = Split Number(x=w1707) -> (hi(x)=w1693:u8, lo(x)=w1692:u8)
            n300 = Split Number(x=w1655) -> (hi(x)=w1657:u8, lo(x)=w1656:u8)
            n301 = Add(x=w1668, y=w1661) -> (x+y=w1667:u32)
            n302 = Split Number(x=w1714) -> (hi(x)=w1704:u8, lo(x)=w1703:u8)
            n303 = Split Number(x=w1713) -> (hi(x)=w1702:u8, lo(x)=w1701:u8)
            n304 = Split Number(x=w1712) -> (hi(x)=w1700:u8, lo(x)=w1699:u8)
            n305 = Build Array "BD 1 A Stack"(w1660, w1659) -> (w1689:u8[])
            n306 = Build Array "BD 2 nu Stack"(w1697, w1696, w1695, w1694, w1693, w1692) -> (w1691:u8[])
            n307 = Build Array "BD 2 A Stack"(w1657, w1656) -> (w1688:u8[])
            n308 = Build Array "BD 1 nu Stack"(w1704, w1703, w1702, w1701, w1700, w1699) -> (w1698:u8[])
            n309 = case shown="2" w1705 {
              tunnel: [w1781 w1784] -> w1687
              tunnel: [u8 10 u8 4] -> w1690
              tunnel: "Swap F1 and F2" -> [w1782 w1784]
              frame #0 {
                # "F2"
                n310 = Not(x=w1782) -> (.not. x?=w1781:bool)
              }
              frame #1 {
                # "low chooses F1"
                # "F1"
              }
            }
            n311 = case "If FPGA is controlling (toggling) RF synth" shown="True" w1686 {
              tunnel: w1698 -> [_ w1734]
              tunnel: w1691 -> [_ w1733]
              tunnel: w1690 -> [_ w1732]
              tunnel: w1689 -> [_ w1731]
              tunnel: w1688 -> [_ w1730]
              frame #0 {
              }
              frame #1 {
                # "Write next amp.\n(wait until beginning of next loop iteration to update)"
                n312 = flat-sequence "Update the next F1 and F2 frequency value (the actual frequency won't change until FSK is switched).\nThen load the next amplitude value into buffer, but don't update it until the next cycle." {
                  tunnel: w1734 -> [w1737]
                  tunnel: w1733 -> [w1736]
                  tunnel: w1732 -> [w1735]
                  tunnel: w1731 -> [w1774]
                  tunnel: w1730 -> [w1773]
                  frame #0 {
                    n313 = for {
                      tunnel: w1737 -> [w1743] mode=indexing
                      tunnel: w1736 -> [w1742] mode=indexing
                      tunnel: w1735 -> [w1740]
                      i -> [w1741]
                      # "Write next freq."
                      n314 = To Unsigned Byte Integer(number=w1741) -> (unsigned 8bit integer=w1738:u8)
                      n315 = Add(x=w1740, y=w1738) -> (x+y=w1739:u8)
                      n316 = call "write to RF synth bd.vi"("Address Byte"=w1739, "BD 2 Byte"=w1742, "BD 1 Byte"=w1743) -> ()
                    }
                  }
                  frame #1 {
                    # "send udclk high"
                    n317 = xnode "FPGA I/O Node"("Connector1/DIO30"=TRUE ("Connector1/DIO15")) -> ()  [unwired: 1 in, 1 out]
                  }
                  frame #2 {
                    n318 = xnode "FPGA I/O Node"("Connector1/DIO30"=FALSE ("Connector1/DIO15")) -> ()  [unwired: 1 in, 1 out]
                  }
                  frame #3 {
                    n319 = for {
                      tunnel: w1774 -> [w1780] mode=indexing
                      tunnel: w1773 -> [w1779] mode=indexing
                      tunnel: u8 33 -> [w1777]
                      i -> [w1778]
                      n320 = To Unsigned Byte Integer(number=w1778) -> (unsigned 8bit integer=w1775:u8)
                      n321 = Add(x=w1777, y=w1775) -> (x+y=w1776:u8)
                      n322 = call "write to RF synth bd.vi"("Address Byte"=w1776, "BD 2 Byte"=w1779, "BD 1 Byte"=w1780) -> ()
                    }
                  }
                }
              }
            }
          }
        }
      }
    }
  }
  n323 = while "Control APD data integration - stream to host" {
    shift-right: [w1878] -> _
    shift-left: w1 -> [w1883]
    stop <- FALSE stop-if-true
    n324 = flat-sequence {
      tunnel: w1883 -> [w1885]
      tunnel: [w1886] -> w1881
      tunnel: [w1885] -> w1879
      tunnel: [w1894] -> w1882
      tunnel: w1881 -> [w1894]
      tunnel: [w1893] -> w1880
      tunnel: w1879 -> [w1893]
      tunnel: [w1892] -> w1877
      tunnel: [w1891] -> w1876
      tunnel: [w1918] -> w1878
      tunnel: w1882 -> [w1943]
      tunnel: w1880 -> [w1940]
      tunnel: w1877 -> [w1911]
      tunnel: w1876 -> [w1910]
      frame #0 {
        n325 = call "Loop Timer6"("Count(Ticks)"=w1885) -> ("Tick Count(Ticks)"=w1886:u32)
      }
      frame #1 {
        n326 = flat-sequence {
          tunnel: [w1895] -> w1890
          tunnel: w1890 -> [w1898]
          tunnel: [w1900] -> w1889
          tunnel: [w1899] -> w1888
          tunnel: [w1898] -> w1887
          tunnel: [w1906] -> w1891
          tunnel: [w1907] -> w1892
          tunnel: w1889 -> [w1907]
          tunnel: w1888 -> [w1906]
          tunnel: w1887 -> [w1905]
          frame #0 {
            n327 = feedback #31(FALSE) -> (w1896:bool)
            "APD out state" <- w1896
            n328 = Not(x=w1896) -> (.not. x?=w1895:bool)
          }
          frame #1 {
            n329 = local read "APD 1 Counts 1"() -> (w1904:u32)
            n330 = local read "APD 1 Counts 0"() -> (w1903:u32)
            n331 = local read "APD 2 Counts 1"() -> (w1902:u32)
            n332 = local read "APD 2 Counts 0"() -> (w1901:u32)
            n333 = Select(t=w1904, s=w1898, f=w1903) -> (s? t:f=w1900:u32)
            n334 = Select(t=w1902, s=w1898, f=w1901) -> (s? t:f=w1899:u32)
          }
          frame #2 {
            n335 = case shown="False" w1905 {
              frame #0 {
                w1908 = u32 0 ("APD 1 Counts 0")
                n336 = local write "APD 1 Counts 0"(w1908) -> ()
                n337 = local write "APD 2 Counts 0"(w1908) -> ()
              }
              frame #1 {
                w1909 = u32 0 ("APD 1 Counts 1")
                n338 = local write "APD 1 Counts 1"(w1909) -> ()
                n339 = local write "APD 2 Counts 1"(w1909) -> ()
              }
            }
          }
        }
      }
      frame #2 {
        n340 = feedback #32(w1943) -> (w1942:u32)
        n341 = Subtract(x=w1943, y=w1942) -> (x-y=w1941:u32)
        n342 = Subtract(x=w1941, y=w1940) -> (x-y=w1934:u32)
        n343 = case shown="True" "APD to FIFO" {
          tunnel: w1911 -> [_ w1970]
          tunnel: w1910 -> [_ w1968]
          frame #0 {
          }
          frame #1 {
            n344 = flat-sequence {
              tunnel: 0 ("Timeout") -> [w1972]
              tunnel: w1970 -> [w1973]
              tunnel: [w1972] -> w1969
              tunnel: w1969 -> [w2000]
              tunnel: w1968 -> [w1999]
              frame #0 {
                n345 = xnode ("FIFO Write")("Element"=w1973, "Timeout"=w1972) -> ()  [unwired: 1 in, 2 out]
              }
              frame #1 {
                n346 = xnode ("FIFO Write")("Element"=w1999, "Timeout"=w2000) -> ()  [unwired: 1 in, 2 out]
              }
            }
          }
        }
        n347 = Subtract(x="APD Acq Rate Count", y=w1934) -> (x-y=w1919:u32)
        n348 = Greater?(x=w1934, y=u32 0) -> (0:w1936:bool)
        "APD Acq Late?" <- w1936
        n349 = feedback #33(u32 0) -> (w1938:u32)
        n350 = Increment(x=w1938) -> (x+1=w1937:u32)
        n351 = Select(t=w1937, s=w1936, f=w1938) -> (s? t:f=w1935:u32)
        "APD Acq Late Counter" <- w1935
        n352 = Boolean To (0,1)(Boolean="+ phase (APD Acq)") -> (0, 1=w1915:i16)
        n353 = Multiply(x=w1915, y="Phase Count Adjustment (APD Acq)") -> (x*y=w1912:i16)
        n354 = Add(x=w1919, y=w1912) -> (x+y=w1918:u32)
        n355 = feedback #34(i16 0) -> (w1917:i16)
        n356 = Subtract(x=w1917, y=w1912) -> (x-y=w1914:i16)
        "APD Acq Relative Phase" <- w1914
        n357 = To Word Integer(number=w1911) -> (16bit integer=w1927:i16)
        n358 = To Word Integer(number=w1910) -> (16bit integer=w1928:i16)
        n359 = Multiply(x="APD 1 AO scale factor", y=w1927) -> (x*y=w1926:i16)
        n360 = Multiply(x="APD 2 AO scale factor", y=w1928) -> (x*y=w1925:i16)
        n361 = Add(x="APD 1 AO offset", y=w1926) -> (x+y=w1924:i16)
        n362 = Add(x=w1925, y="APD 2 AO offset") -> (x+y=w1922:i16)
        n363 = xnode "FPGA I/O Node"("Connector0/AO6"=w1924, "Connector0/AO7"=w1922) -> ()  [unwired: 2 in, 2 out]
      }
    }
  }
  n364 = while "MCL stage control" {
    shift-right: [w2041] -> _
    shift-left: w1 -> [w2044]
    shift-right: [w2034] -> _
    shift-left: w5 -> [w2031]
    shift-right: [w2033] -> _
    shift-left: w4 -> [w2029]
    i -> [w2028]
    stop <- FALSE stop-if-true
    n365 = flat-sequence {
      tunnel: w2044 -> [w2048]
      tunnel: [w2049] -> w2040
      tunnel: [w2048] -> w2038
      tunnel: [w2047] -> w2032
      tunnel: w2031 -> [w2047]
      tunnel: [w2046] -> w2030
      tunnel: w2029 -> [w2046]
      tunnel: w2040 -> [w2053]
      tunnel: [w2053] -> w2039
      tunnel: w2038 -> [w2052]
      tunnel: [w2052] -> w2037
      tunnel: w2032 -> [w2051]
      tunnel: w2030 -> [w2050]
      tunnel: [w2051] -> w2027
      tunnel: [w2050] -> w2026
      tunnel: w2039 -> [w2087]
      tunnel: w2037 -> [w2086]
      tunnel: [w2087] -> w2043
      tunnel: [w2086] -> w2042
      tunnel: [w2085] -> w2036
      tunnel: [w2084] -> w2035
      tunnel: w2027 -> [w2079]
      tunnel: w2026 -> [w2078]
      tunnel: [w2151] -> w2041
      tunnel: w2043 -> [w2165]
      tunnel: w2042 -> [w2162]
      tunnel: w2036 -> [w2154]
      tunnel: w2035 -> [w2153]
      tunnel: [w2154] -> w2034
      tunnel: [w2153] -> w2033
      frame #0 {
        n366 = call "Loop Timer5"("Count(Ticks)"=w2048) -> ("Tick Count(Ticks)"=w2049:u32)
      }
      frame #1 {
        n367 = xnode "FPGA I/O Node"("Connector0/AO1"=w2051, "Connector0/AO2"=w2050) -> ()  [unwired: 2 in, 2 out]
      }
      frame #2 {
        n368 = local read "Scanning MCL"() -> (w2099:bool)
        n369 = Or(x=w2099, y="Start scan (MCL)") -> (x .or. y?=w2094:bool)
        n370 = Not(x="Abort scan (MCL)") -> (.not. x?=w2092:bool)
        n371 = And(x=w2092, y=w2094) -> (x .and. y?=w2091:bool)
        n372 = case "Raster scan" shown="True" w2091 {
          tunnel: [w2100 w2143] -> w2096
          tunnel: "Start scan (MCL)" -> [_ w2128]
          tunnel: [w2100 w2104] -> w2080
          frame #0 {
            w2100 = i16 0
            n373 = local write "Scanning MCL"(FALSE ("scanning")) -> ()
          }
          frame #1 {
            w2114 = i16 0
            w2113 = u64 0
            # "scan incr."
            # "freq. incr. mult."
            # "count steps"
            # "count number of cycles"
            n374 = feedback #35(w2113) -> (w2140:u64)
            n375 = Select(t=w2113, s=w2128, f=w2140) -> (s? t:f=w2142:u64)
            n376 = Increment(x=w2142) -> (x+1=w2139:u64)
            n377 = Greater?(x="Cycles per step (MCL)", y=w2139) -> (0:w2123:bool)
            n378 = Select(t=w2139, s=w2123, f=w2113) -> (s? t:f=w2138:u64)
            n379 = feedback #36(w2113) -> (w2137:u64)
            n380 = Select(t=w2113, s=w2128, f=w2137) -> (s? t:f=w2132:u64)
            n381 = Increment(x=w2132) -> (x+1=w2136:u64)
            n382 = Add(x="Scan steps (MCL)", y="Scan steps (MCL)") -> (x+y=w2135:u64)
            n383 = Select(t=w2132, s=w2123, f=w2136) -> (s? t:f=w2118:u64)
            n384 = Greater?(x=w2135, y=w2118) -> (0:w2117:bool)
            n385 = Select(t=w2118, s=w2117, f=w2113) -> (s? t:f=w2133:u64)
            n386 = Equal?(x="Scan steps (MCL)", y=w2118) -> (x = y?=w2122:bool)
            n387 = Greater?(x="Scan steps (MCL)", y=w2132) -> (0:w2131:bool)
            n388 = feedback #37(w2114) -> (w2134:i16)
            n389 = Select(t=w2114, s=w2128, f=w2134) -> (s? t:f=w2120:i16)
            n390 = Increment(x=w2120) -> (x+1=w2130:i16)
            n391 = Decrement(x=w2120) -> (x-1=w2129:i16)
            n392 = Select(t=w2130, s=w2131, f=w2129) -> (s? t:f=w2121:i16)
            n393 = Select(t=w2120, s=w2122, f=w2121) -> (s? t:f=w2119:i16)
            n394 = Select(t=w2120, s=w2123, f=w2119) -> (s? t:f=w2115:i16)
            n395 = Select(t=w2115, s=w2117, f=w2114) -> (s? t:f=w2116:i16)
            n396 = feedback #38(w2113) -> (w2127:u64)
            n397 = Select(t=w2113, s=w2128, f=w2127) -> (s? t:f=w2102:u64)
            n398 = Increment(x=w2102) -> (x+1=w2124:u64)
            n399 = Select(t=w2102, s=w2117, f=w2124) -> (s? t:f=w2103:u64)
            n400 = Greater?(x="Number of scans (MCL)", y=w2103) -> (0:w2110:bool)
            n401 = Multiply(x="Scan freq.  increment (MCL)", y=w2120) -> (x*y=w2143:i16)
            n402 = Select(t=TRUE, s="Cont. Scan (MCL)", f=w2110) -> (s? t:f=w2109:bool)
            "Scanning MCL" <- w2109
            n403 = Select(t=w2103, s=w2109, f=w2113) -> (s? t:f=w2125:u64)
            n404 = Increment(x=w2103) -> (x+1=→"Scan I (MCL)":u64)
            n405 = To Word Integer(number=w2102) -> (16bit integer=w2105:i16)
            n406 = Multiply(x=w2105, y="Scan freq.  increment (MCL)") -> (x*y=w2104:i16)
          }
        }
        n407 = Select(t=w2080, s="1D or 2D Scan?", f=i16 0) -> (s? t:f=w2081:i16)
        n408 = Select(t=w2081, s="MCL Scan Axis", f=w2096) -> (s? t:f=w2095:i16)
        n409 = Select(t=w2096, s="MCL Scan Axis", f=w2081) -> (s? t:f=w2097:i16)
        n410 = Add(x=w2095, y="AO2") -> (x+y=w2084:i16)
        n411 = Add(x="AO1", y=w2097) -> (x+y=w2085:i16)
        "AO1 2" <- w2079
        "AO2 2" <- w2078
      }
      frame #3 {
        n412 = feedback #39(w2165) -> (w2164:u32)
        n413 = Boolean To (0,1)(Boolean="+ phase (MCL)") -> (0, 1=w2149:i16)
        n414 = Subtract(x=w2165, y=w2164) -> (x-y=w2163:u32)
        n415 = Multiply(x=w2149, y="Phase count adjustment (MCL)") -> (x*y=w2145:i16)
        n416 = Subtract(x=w2163, y=w2162) -> (x-y=w2160:u32)
        n417 = Subtract(x="MCL count", y=w2160) -> (x-y=w2147:u32)
        n418 = feedback #40(i16 0) -> (w2146:i16)
        n419 = Subtract(x=w2146, y=w2145) -> (x-y=w2144:i16)
        "MCL Relative Phase" <- w2144
        n420 = Greater?(x=w2160, y=u32 0) -> (0:w2159:bool)
        "MCL Late?" <- w2159
        n421 = Add(x=w2147, y=w2145) -> (x+y=w2151:u32)
        n422 = feedback #41(u32 0) -> (w2157:u32)
        n423 = Increment(x=w2157) -> (x+1=w2156:u32)
        n424 = Select(t=w2156, s=w2159, f=w2157) -> (s? t:f=w2158:u32)
        "MCL Late Counter" <- w2158
      }
    }
    "Numeric" <- w2028
  }
  n425 = while "RF box board direct communication loop" {
    tunnel: w1 -> [_]
    stop <- FALSE stop-if-true
    n426 = case "Whether to use direct communication method (only use one method at a time)" shown="True" "Direct RF Box \nCommunication" {
      frame #0 {
      }
      frame #1 {
        n427 = case shown="True" "Update Data" {
          frame #0 {
          }
          frame #1 {
            n428 = flat-sequence {
              frame #0 {
                n429 = First Call?() -> (First Call?: T/F=w2170:bool)
                n430 = case shown="True" w2170 {
                  frame #0 {
                  }
                  frame #1 {
                    # "If first time data updated, be sure to set WR high\nbefore setting data and address bits."
                    n431 = flat-sequence {
                      frame #0 {
                        n432 = xnode "FPGA I/O Node"("Connector1/DIO15"=TRUE) -> ()  [unwired: 1 in, 1 out]
                      }
                      frame #1 {
                        n433 = call "Wait"("Count(Ticks)"=u8 40 ("DO Delay 3 (Ticks)")) -> ()  [unwired: 1 out]
                      }
                    }
                  }
                }
              }
              frame #1 {
                n434 = Number To Boolean Array(number="Address") -> (Boolean array=w2232:bool[])
                n435 = Number To Boolean Array(number="Data BD 1") -> (Boolean array=w2233:bool[])
                n436 = Number To Boolean Array(number="Data BD 2") -> (Boolean array=w2202:bool[])
                n437 = Index Array(array=w2233, index=7) -> (element=w2217:bool)
                n438 = Index Array(array=w2233, index=6) -> (element=w2216:bool)
                n439 = Index Array(array=w2233, index=5) -> (element=w2215:bool)
                n440 = Index Array(array=w2233, index=4) -> (element=w2214:bool)
                n441 = Index Array(array=w2233, index=3) -> (element=w2213:bool)
                n442 = Index Array(array=w2233, index=2) -> (element=w2212:bool)
                n443 = Index Array(array=w2233, index=1) -> (element=w2211:bool)
                n444 = Index Array(array=w2233, index=0) -> (element=w2210:bool)
                n445 = Index Array(array=w2232, index=5) -> (element=w2209:bool)
                n446 = Index Array(array=w2232, index=4) -> (element=w2208:bool)
                n447 = Index Array(array=w2232, index=3) -> (element=w2207:bool)
                n448 = Index Array(array=w2232, index=2) -> (element=w2206:bool)
                n449 = Index Array(array=w2232, index=1) -> (element=w2205:bool)
                n450 = Index Array(array=w2232, index=0) -> (element=w2204:bool)
                n451 = Index Array(array=w2202, index=7) -> (element=w2193:bool)
                n452 = Index Array(array=w2202, index=6) -> (element=w2192:bool)
                n453 = Index Array(array=w2202, index=5) -> (element=w2191:bool)
                n454 = Index Array(array=w2202, index=4) -> (element=w2190:bool)
                n455 = Index Array(array=w2202, index=3) -> (element=w2189:bool)
                n456 = Index Array(array=w2202, index=2) -> (element=w2188:bool)
                n457 = Index Array(array=w2202, index=1) -> (element=w2187:bool)
                n458 = Index Array(array=w2202, index=0) -> (element=w2186:bool)
                n459 = xnode "FPGA I/O Node"("Connector1/DIO0"=w2217, "Connector1/DIO1"=w2216, "Connector1/DIO2"=w2215, "Connector1/DIO3"=w2214, "Connector1/DIO4"=w2213, "Connector1/DIO5"=w2212, "Connector1/DIO6"=w2211, "Connector1/DIO7"=w2210, "Connector1/DIO8"=w2209, "Connector1/DIO9"=w2208, "Connector1/DIO10"=w2207, "Connector1/DIO11"=w2206, "Connector1/DIO12"=w2205, "Connector1/DIO13"=w2204, "Connector1/DIO20"=w2193, "Connector1/DIO21"=w2192, "Connector1/DIO22"=w2191, "Connector1/DIO23"=w2190, "Connector1/DIO24"=w2189, "Connector1/DIO25"=w2188, "Connector1/DIO26"=w2187, "Connector1/DIO27"=w2186) -> ()  [unwired: 22 in, 22 out]
              }
              frame #2 {
                # "wait and then apply write signal"
                n460 = call "Wait2"("Count(Ticks)"=u8 40 ("DO Delay 1 (Ticks)")) -> ()  [unwired: 1 out]
              }
              frame #3 {
                # "sending bit low writes data to board buffer"
                n461 = xnode "FPGA I/O Node"("Connector1/DIO15"=FALSE) -> ()  [unwired: 1 in, 1 out]
              }
              frame #4 {
                # "wait then return write signal"
                n462 = call "Wait3"("Count(Ticks)"=u8 40 ("DO Delay 2 (Ticks)")) -> ()  [unwired: 1 out]
              }
              frame #5 {
                # "sending bit high makes ready to\nwrite more data"
                n463 = xnode "FPGA I/O Node"("Connector1/DIO15"=TRUE) -> ()  [unwired: 1 in, 1 out]
              }
            }
          }
        }
      }
    }
  }
  n464 = node-c288(w2) -> ()
